vi "get all FPGA CD resources.vi"(7 "Show":T4, 8 "error in (no error)":errorcluster, 11 "Item Ref in":T1 format="%.0x") -> (0 "error out":errorcluster, 2 "fpga resources":cluster{"fpga cd":T1, "resource":T2}[](array[cluster]) {"fpga cd" format="%.0x"}, 3 "Item Ref out":T1 format="%.0x")   [LabVIEW 2016, in "FPGA Resource Manager System Definition.lvlib"]
uses:
  FPGA Resource Manager System Definition.lvlib
  <vilib>/NI Veristand/Custom Device API/Custom Device Item Ref.ctl
  viz_show.ctl
  FPGA-Addon/Source/System Explorer/SubVIs/fpga resource.ctl
  FPGA-Addon/Source/System Explorer/SubVIs/Channel Type.ctl
  <vilib>/NI VeriStand/Custom Device API/Custom Device API.lvlib
  FPGA-Addon/Source/System Explorer/FPGA Addon System Explorer.lvlib
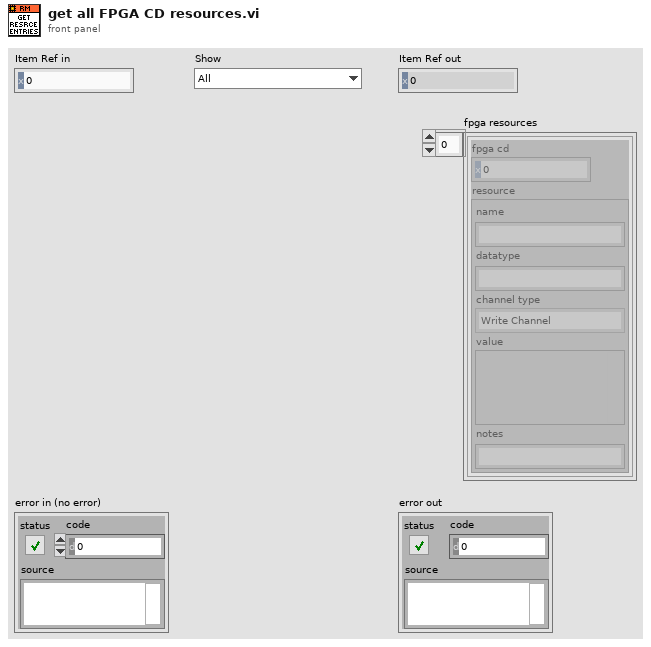
[diagram p1: front panel]
types:
  T1 = typedef "Custom Device API.lvlib/Custom Device Item Ref.ctl" = u64
  T2 = typedef "FPGA Addon System Explorer.lvlib/fpga resource.ctl" = cluster{"name":string, "datatype":string, "channel type":T3, "value":variant, "notes":string}
  T3 = typedef "FPGA Addon System Explorer.lvlib/Channel Type.ctl" = enum16{"Write Channel", "Read Channel", "Write Waveform", "Read Waveform"}
  T4 = typedef "FPGA Resource Manager System Definition.lvlib/viz_show.ctl" = enum16{"All", "Mapped", "Unmapped"}
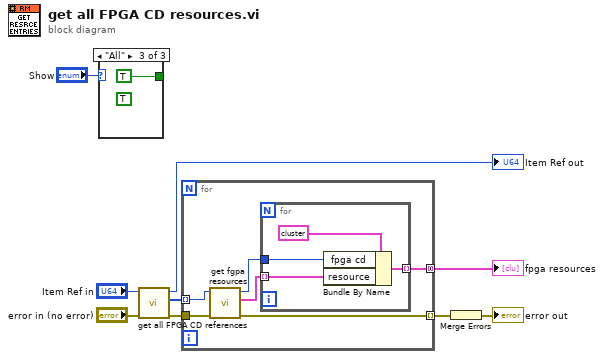
[diagram p0: block diagram]
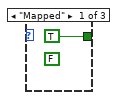
[diagram p2: hidden frame]
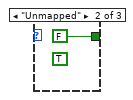
[diagram p3: hidden frame]
diagram:
  n1 = case shown="\"All\"" "Show" {
    tunnel: [TRUE FALSE TRUE] -> _
    frame "Mapped" {
      (unwired) FALSE
    }
    frame "Unmapped" {
      (unwired) TRUE
    }
    frame "All" {
      (unwired) TRUE
    }
  }
  n2 = call "get all FPGA CD references.vi"("error in (no error)"="error in (no error)", "Item Ref in"="Item Ref in") -> ("error out"=w3:errorcluster, "RM Server refs out"=w5:T1[], "Item Ref out"=→"Item Ref out":T1)  [unwired: 7 in]
  n3 = for {
    tunnel: w3 -> [w18]
    tunnel: w5 -> [w16] mode=indexing
    tunnel: [w17] -> w9 mode=indexing
    tunnel: [w13] -> w1 mode=concatenating
    n4 = call "get fgpa resources.vi"("error in (no error)"=w18, "Item Ref in"=w16) -> ("error out"=w17:errorcluster, "get fpga resources"=w15:T2[], "Item Ref out"=w14:T1)  [unwired: 6 in, 1 out]
    n5 = for {
      tunnel: w15 -> [w22] mode=indexing
      tunnel: w14 -> [w21]
      tunnel: [w19] -> w13 mode=indexing
      n6 = Bundle By Name(cluster=cluster{"fpga cd":T1, "resource":T2} {"fpga cd"=0, "resource"={"name"="", "datatype"="", "channel type"=enum."Write Channel", "value"=variant, "notes"=""}}, "fpga cd"=w21, "resource"=w22) -> (w19:cluster{"fpga cd":T1, "resource":T2})
    }
  }
  "fpga resources" <- w1
  n7 = Merge Errors(w9) -> (→"error out":errorcluster)
